vi "Test Android Sensor.vi"() -> ()   [LabVIEW 2011]
uses:
  <vilib>/TOOLS FOR SMART MINDS/SCCT/Publisher/Publisher.lvclass
  <vilib>/TOOLS FOR SMART MINDS/SCCT/Publisher/publishData_Message.vi
panel:
  out "port":u16
  in  "milliseconds to wait 2":u32=10
  in  "milliseconds to wait":u32=990
  out "activeSubscribersAddress":string[][](array[string])
  in  "stop 2":bool
  out "s? t:f":dbl
  in  "stop":bool
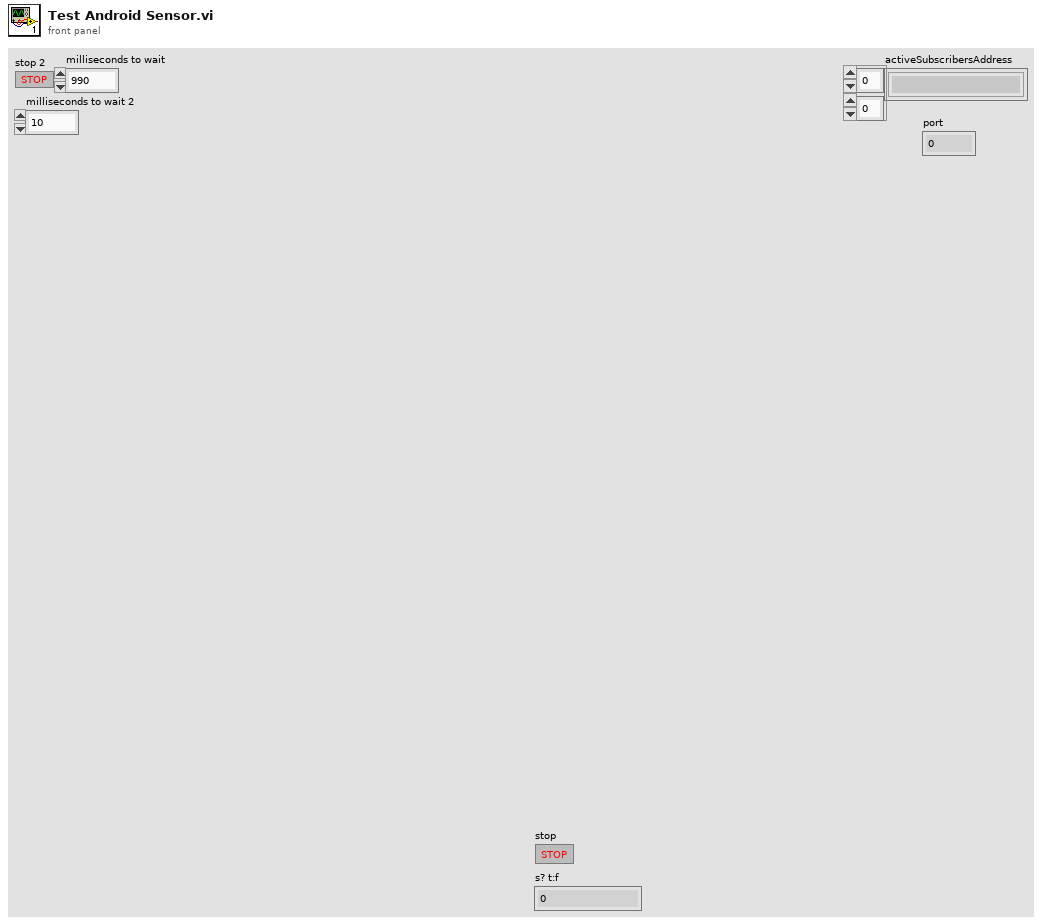
[diagram p1: front panel]
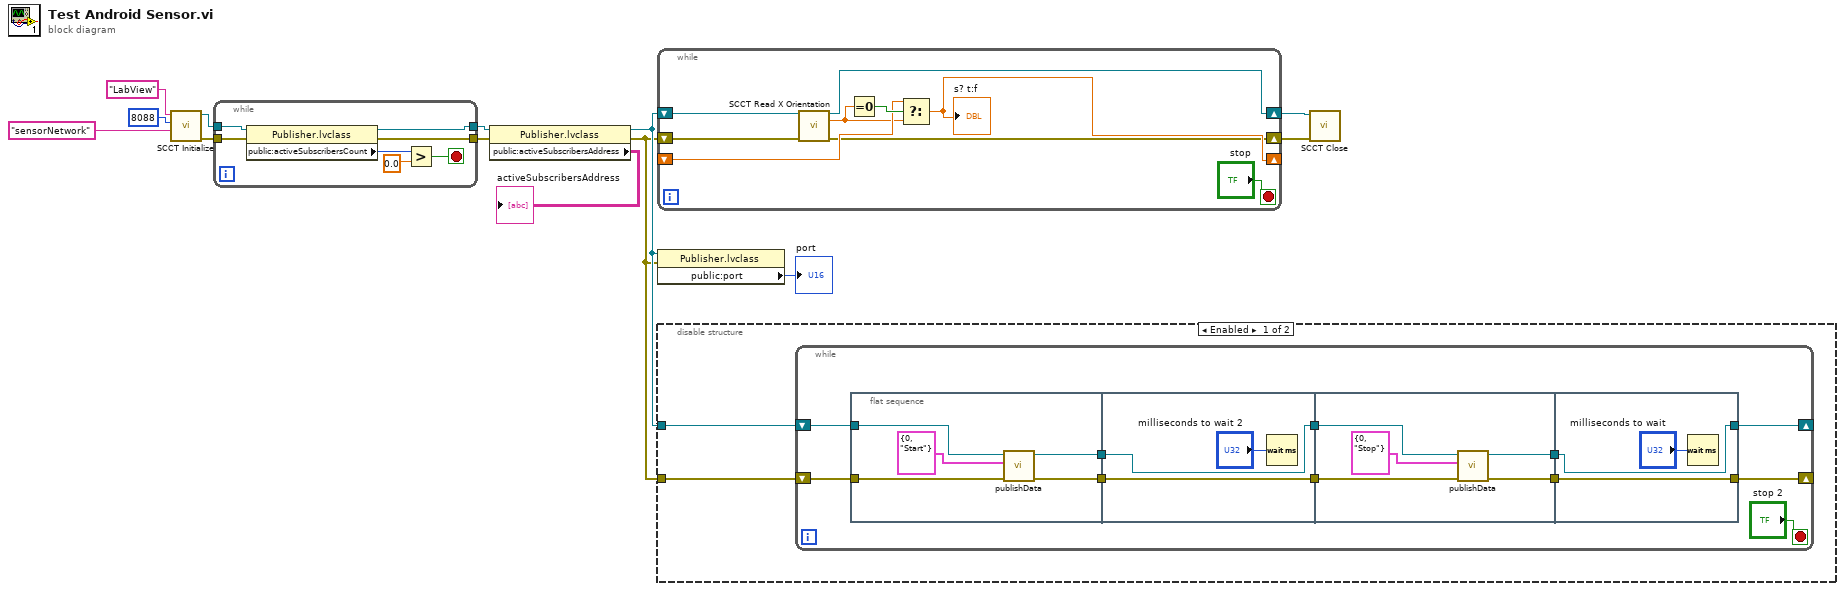
[diagram p0: block diagram]
diagram:
  n1 = call "SCCT Initialize.vi"("API-Key"="sensorNetwork", "publisherPort"=u16 8088, "description"="LabView") -> ("error out"=w7:errorcluster, "publisher out"=w8:refnum<class "Publisher.lvclass">)  [unwired: 7 in]
  n2 = while {
    tunnel: w8 -> [w20]
    tunnel: w7 -> [w19]
    tunnel: [w18] -> w3
    tunnel: [w17] -> w2
    stop <- w14 stop-if-true
    n3 = property class="Publisher.lvclass"(reference=w20, error in=w19) -> (reference out=w18:refnum<class "Publisher.lvclass">, error out=w17:errorcluster, "public:activeSubscribersCount"=w15:i32)
    n4 = Greater?(x=w15, y=0.0) -> (0:w14:bool)
  }
  n5 = property class="Publisher.lvclass"(reference=w3, error in=w2) -> (reference out=w6:refnum<class "Publisher.lvclass">, error out=w5:errorcluster, "public:activeSubscribersAddress"=→"activeSubscribersAddress":string[][])
  n6 = while {
    shift-right: [w24] -> w13
    shift-left: w6 -> [w21]
    shift-right: [w23] -> w12
    shift-left: w5 -> [w25]
    shift-right: [w27] -> _
    shift-left: _ -> [w26]
    stop <- "stop" stop-if-true
    n7 = call "SCCT Read X Orientation.vi"("Publisher In"=w21, "input cluster"=w25) -> ("Publisher Out"=w24:refnum<class "Publisher.lvclass">, "X Orientation"=w22:dbl, "error out 2"=w23:errorcluster)  [unwired: 9 in, 2 out]
    n8 = Equal To 0?(x=w22) -> (x = 0?=w28:bool)
    n9 = Select(t=w26, s=w28, f=w22) -> (s? t:f=w27:dbl)
    "s? t:f" <- w27
  }
  n10 = property class="Publisher.lvclass"(reference=w6, error in=w5) -> ("public:port"=→"port":u16)  [unwired: 2 out]
  n11 = disable-structure shown="Enabled" {
    disable-tunnel: w6 -> [w31 _]
    disable-tunnel: w5 -> [w30 _]
    frame Enabled {
      n12 = while {
        shift-right: [w34] -> _
        shift-left: w31 -> [w36]
        shift-right: [w33] -> _
        shift-left: w30 -> [w35]
        stop <- "stop 2" stop-if-true
        n13 = flat-sequence {
          tunnel: w36 -> [w46]
          tunnel: w35 -> [w45]
          tunnel: [w44] -> w42
          tunnel: [w43] -> w41
          tunnel: w42 -> [w50]
          tunnel: w41 -> [w49]
          tunnel: [w50] -> w40
          tunnel: [w49] -> w39
          tunnel: w40 -> [w54]
          tunnel: w39 -> [w52]
          tunnel: [w53] -> w38
          tunnel: [w51] -> w37
          tunnel: [w57] -> w33
          tunnel: [w58] -> w34
          tunnel: w38 -> [w58]
          tunnel: w37 -> [w57]
          frame #0 {
            n14 = call-poly <vilib>:"publishData.vi"("error in (no error)"=w45, "value"=cluster{"code":i32, "description":string} {"code"=0, "description"="Start"}, "publisher in"=w46) -> ("error out"=w43:errorcluster, "publisher out"=w44:refnum<class "Publisher.lvclass">)  [unwired: 7 in]
          }
          frame #1 {
            n15 = Wait (ms)(milliseconds to wait="milliseconds to wait 2") -> ()  [unwired: 1 out]
          }
          frame #2 {
            n16 = call-poly <vilib>:"publishData.vi"("error in (no error)"=w52, "value"=cluster{"code":i32, "description":string} {"code"=0, "description"="Stop"} ("value 2"), "publisher in"=w54) -> ("error out"=w51:errorcluster, "publisher out"=w53:refnum<class "Publisher.lvclass">)  [unwired: 7 in]
          }
          frame #3 {
            n17 = Wait (ms)(milliseconds to wait="milliseconds to wait") -> ()  [unwired: 1 out]
          }
        }
      }
    }
    frame Disabled {
    }
  }
  n18 = call "SCCT Close.vi"("error in (no error)"=w12, "Publisher In"=w13) -> ()  [unwired: 9 in, 1 out]
